vi "Cumulative StatisticalParamets.vi"(6 "N":i32, 8 "error in (no error)":errorcluster, 9 "Measurement Data":dbl[](array[numeric]), 10 "DataIn":T2(array[cluster]), 11 "Initialization Data":T1={"Measurement-ID"=[0, 1, 2, 3, 4, 5], "Measurement Names"=["a", "b", "C", "D", "E"], "NominalValues"=[1.5, 2.3], "LSL"=[1.0, 1.8, 2.0, 2.6, 2.7], "USL"=[2.0, 2.8, 3.2, 3.4, 3.8], "LCL"=[1.0, 1.8], "UCL"=[2.0, 2.8]}) -> (0 "error out":errorcluster, 2 "DataOut":T2(array[cluster]), 3 "Statistical Parameters":string[][](array[string]))   [LabVIEW 2019, in "Zen Analytics.lvlib" / "Zen Analytics.lvclass"]
uses:
  Zen Analytics.lvclass
types:
  T1 = cluster{"Measurement-ID":i32[], "Measurement Names":string[], "NominalValues":dbl[], "LSL":dbl[], "USL":dbl[], "LCL":dbl[], "UCL":dbl[]}
  T2 = cluster{"SumOfSquareOfData":dbl, "SumOfMeasurementData":dbl, "N ":u32}[]
  T3 = cluster{"SumOfSquareOfData":dbl, "SumOfMeasurementData":dbl, "N ":u32}
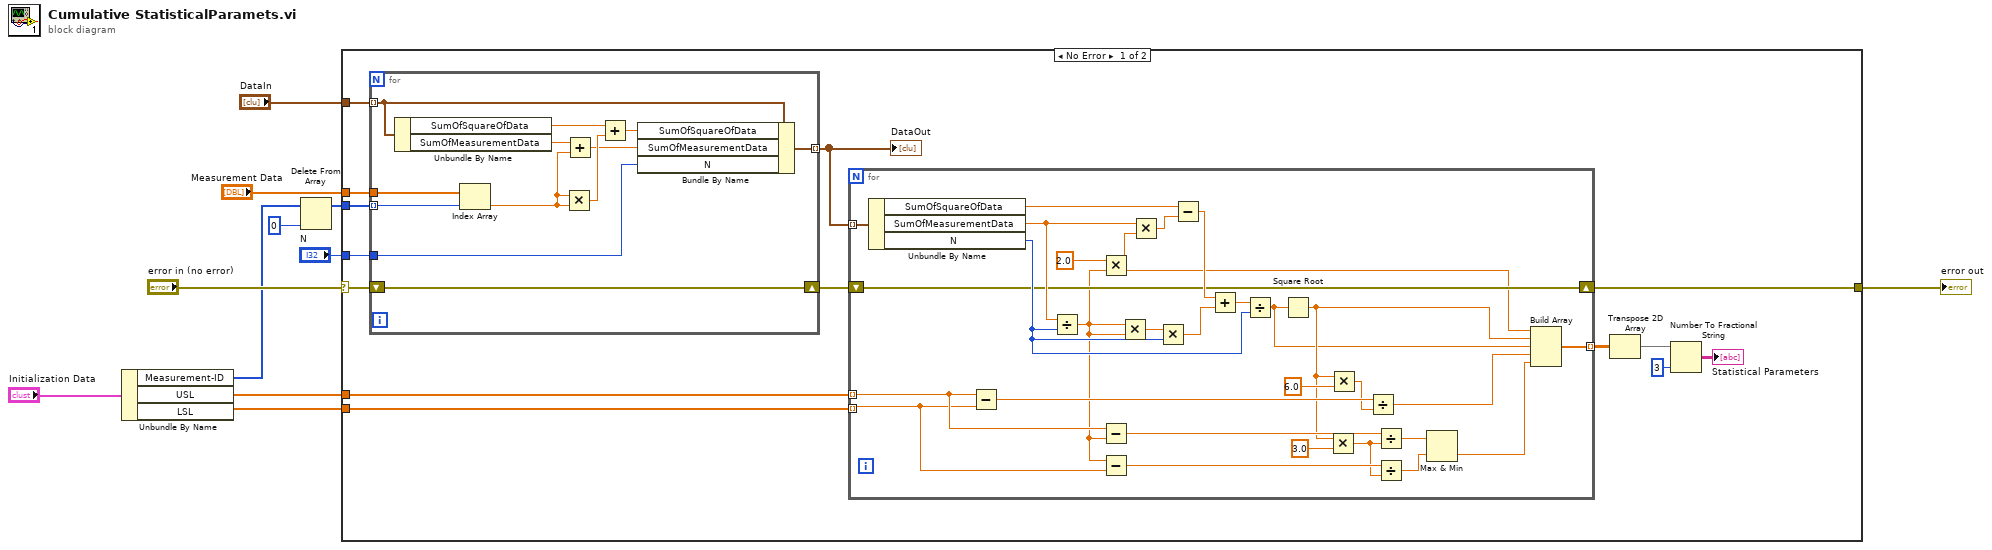
[diagram p0: block diagram]
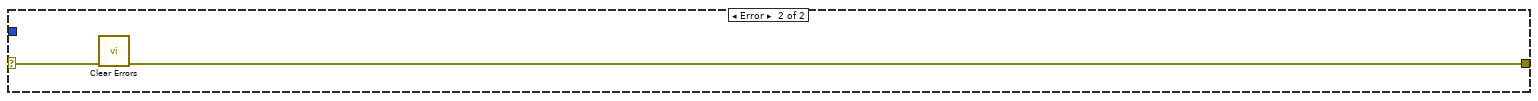
[diagram p2: hidden frame]
diagram:
  n1 = Unbundle By Name("Initialization Data") -> ("Measurement-ID"=w3:i32[], "USL"=w5:dbl[], "LSL"=w4:dbl[])
  n2 = Delete From Array(array=w3, index=0) -> (array with subset deleted=w9:i32[])  [unwired: 1 in, 1 out]
  n3 = case shown="No Error" "error in (no error)" {
    selector: "error in (no error)" -> [w25 w68]
    tunnel: [w16 w67] -> w10
    tunnel: w9 -> [w24 _]
    tunnel: "Measurement Data" -> [w23 _]
    tunnel: "N" -> [w22 _]
    tunnel: "DataIn" -> [w21 _]
    tunnel: w5 -> [w19 _]
    tunnel: w4 -> [w18 _]
    frame No Error {
      n4 = for {
        tunnel: w24 -> [w64] mode=indexing
        shift-right: [w66] -> w17
        shift-left: w25 -> [w66]
        tunnel: w23 -> [w65]
        tunnel: w22 -> [w62]
        tunnel: w21 -> [w63] mode=indexing
        tunnel: [w60] -> w20 mode=indexing
        n5 = Unbundle By Name(w63) -> ("SumOfSquareOfData"=w56:dbl, "SumOfMeasurementData"=w59:dbl)
        n6 = Index Array(array=w65, index=w64) -> (element=w58:dbl)
        n7 = Multiply(x=w58, y=w58) -> (x*y=w61:dbl)
        n8 = Add(x=w59, y=w58) -> (x+y=w57:dbl)
        n9 = Add(x=w56, y=w61) -> (x+y=w55:dbl)
        n10 = Bundle By Name(cluster=w63, "SumOfSquareOfData"=w55, "SumOfMeasurementData"=w57, "N"=w62) -> (w60:T3)
      }
      "DataOut" <- w20
      n11 = for {
        tunnel: w20 -> [w54] mode=indexing
        tunnel: w19 -> [w39] mode=indexing
        tunnel: w18 -> [w38] mode=indexing
        shift-right: [w32] -> w16
        shift-left: w17 -> [w32]
        tunnel: [w26] -> w14 mode=indexing
        n12 = Unbundle By Name(w54) -> ("SumOfSquareOfData"=w53:dbl, "SumOfMeasurementData"=w51:dbl, "N"=w45:u32)
        n13 = Subtract(x=w39, y=w38) -> (x-y=w42:dbl)
        n14 = Divide(x=w51, y=w45) -> (x/y=w31:dbl)
        n15 = Multiply(x=2.0 ("y"), y=w31) -> (x*y=w52:dbl)
        n16 = Subtract(x=w39, y=w31) -> (x-y=w37:dbl)
        n17 = Subtract(x=w31, y=w38) -> (x-y=w36:dbl)
        n18 = Multiply(x=w31, y=w31) -> (x*y=w48:dbl)
        n19 = Multiply(x=w51, y=w52) -> (x*y=w50:dbl)
        n20 = Multiply(x=w48, y=w45) -> (x*y=w47:dbl)
        n21 = Subtract(x=w53, y=w50) -> (x-y=w49:dbl)
        n22 = Add(x=w49, y=w47) -> (x+y=w46:dbl)
        n23 = Divide(x=w46, y=w45) -> (x/y=w29:dbl)
        n24 = Square Root(x=w29) -> (sqrt(x)=w30:dbl)
        n25 = Multiply(x=w30, y=3.0) -> (x*y=w35:dbl)
        n26 = Multiply(x=w30, y=6.0) -> (x*y=w41:dbl)
        n27 = Divide(x=w42, y=w41) -> (x/y=w28:dbl)
        n28 = Divide(x=w37, y=w35) -> (x/y=w34:dbl)
        n29 = Divide(x=w36, y=w35) -> (x/y=w33:dbl)
        n30 = Max & Min(x=w34, y=w33) -> (min(x,y)=w27:dbl)  [unwired: 1 out]
        n31 = Build Array(w31, w30, w29, w28, w27) -> (w26:dbl[])
      }
      n32 = Transpose 2D Array(2D array=w14) -> (transposed array=w13:dbl[][])
      n33 = Number To Fractional String(number=w13, precision (6)=i16 3) -> (F-format string=→"Statistical Parameters":string[][])  [unwired: 2 in]
    }
    frame Error {
      n34 = call <vilib>:"Clear Errors.vi"("error in (no error)"=w68) -> ("error out"=w67:errorcluster)  [unwired: 5 in, 1 out]
    }
  }
  "error out" <- w10
